vi "TallyConsoleErrors.vi"(11 "error log":path) -> (3 "number of errors":i32)   [LabVIEW 2012]
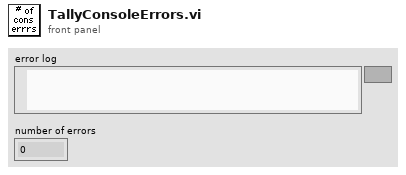
[diagram p1: front panel]
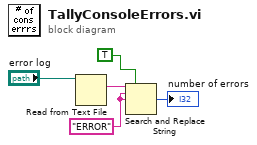
[diagram p0: block diagram]
diagram:
  w2 = "ERROR" ("search string")
  n1 = Read from Text File(file (use dialog)="error log") -> (text=w4:string)  [unwired: 3 in, 3 out]
  n2 = Search and Replace String(replace all?=TRUE ("replace all? (F)"), input string=w4, search string=w2, replace string=w2) -> (number of replacements=→"number of errors":i32)  [unwired: 4 in, 3 out]
